vi "CheckVIStatus.vi"() -> ()   [LabVIEW 2016]
panel:
  out "Locked":path[](array[path])=[path "../../../../examples/Open_GDS/GDS/GOOP3_ActiveObject_Debugger_Open_GDS/Map_class/utils/Map_Delete.vi", path "../../../../examples/Open_GDS/GDS/GOOP3_ActiveObject_Debugger_Open_GDS/Map_class/utils/Map_GetAttributes.vi", path "../../../../examples/Open_GDS/GDS/GOOP3_ActiveObject_Debugger_Open_GDS/Map_class/utils/Map_GetAttributesToModify.vi", path "../../../../examples/Open_GDS/GDS/GOOP3_ActiveObject_Debugger_Open_GDS/Map_class/utils/Map_GetClassAttributes.vi", path "../../../../examples/Open_GDS/GDS/GOOP3_ActiveObject_Debugger_Open_GDS/Map_class/utils/Map_GetClassAttributesToModify.vi", path "../../../../examples/Open_GDS/GDS/GOOP3_ActiveObject_Debugger_Open_GDS/Map_class/utils/Map_GetObjectStatus.vi", path "../../../../examples/Open_GDS/GDS/GOOP3_ActiveObject_Debugger_Open_GDS/Map_class/utils/Map_GOOPKernel.vi", path "../../../../examples/Open_GDS/GDS/GOOP3_ActiveObject_Debugger_Open_GDS/Map_class/utils/Map_New.vi", path "../../../../examples/Open_GDS/GDS/GOOP3_ActiveObject_Debugger_Open_GDS/Map_class/utils/Map_SetModifiedAttributes.vi", path "../../../../examples/Open_GDS/GDS/GOOP3_ActiveObject_Debugger_Open_GDS/Map_class/utils/Map_SetModifiedClassAttributes.vi", path "../../../../examples/Open_GDS/GDS/GOOP3_ActiveObject_Debugger_Open_GDS/Object_class/utils/Object_Delete.vi", path "../../../../examples/Open_GDS/GDS/GOOP3_ActiveObject_Debugger_Open_GDS/Object_class/utils/Object_GetAttributes.vi", path "../../../../examples/Open_GDS/GDS/GOOP3_ActiveObject_Debugger_Open_GDS/Object_class/utils/Object_GetAttributesToModify.vi", path "../../../../examples/Open_GDS/GDS/GOOP3_ActiveObject_Debugger_Open_GDS/Object_class/utils/Object_GetClassAttributes.vi", path "../../../../examples/Open_GDS/GDS/GOOP3_ActiveObject_Debugger_Open_GDS/Object_class/utils/Object_GetObjectStatus.vi", path "../../../../examples/Open_GDS/GDS/GOOP3_ActiveObject_Debugger_Open_GDS/Object_class/utils/Object_GOOPKernel.vi", path "../../../../examples/Open_GDS/GDS/GOOP3_ActiveObject_Debugger_Open_GDS/Object_class/utils/Object_New.vi", path "../../../../examples/Open_GDS/GDS/GOOP3_ActiveObject_Debugger_Open_GDS/Object_class/utils/Object_SetModifiedAttributes.vi", path "../../../../examples/Open_GDS/GDS/GOOP3_ActiveObject_Debugger_Open_GDS/Object_class/utils/Object_SetModifiedClassAttributes.vi", path "../../../../examples/Open_GDS/GDS/GOOP4_CreateObjects_Open_GDS/GOOP4_CreateObjects_Open_GDS.aliases", path "../../../../examples/Open_GDS/GDS/GOOP4_CreateObjects_Open_GDS/GOOP4_CreateObjects_Open_GDS.lvlps", path "../../../../examples/Open_GDS/GDS/GOOP4_CreateObjects_Open_GDS/GOOP4_CreateObjects_Open_GDS.lvproj", path "../../../../examples/Open_GDS/GDS/GOOP4_CreateObjects_Open_GDS/GOOP4_Base_class/utils/GOOP4_Base_GetAttributes.vi", path "../../../../examples/Open_GDS/GDS/GOOP4_CreateObjects_Open_GDS/GOOP4_Base_class/utils/GOOP4_Base_New.vi", path "../../../../examples/Open_GDS/GDS/GOOP4_CreateObjects_Open_GDS/GOOP4_Sub_class/utils/GOOP4_Sub_GetAttributes.vi", path "../../../../examples/Open_GDS/GDS/GOOP4_CreateObjects_Open_GDS/GOOP4_Sub_class/utils/GOOP4_Sub_New.vi", path "../../../../examples/Open_GDS/GDS/InterfaceByViServer/InterfaceByViServer.aliases", path "../../../../examples/Open_GDS/GDS/InterfaceByViServer/InterfaceByViServer.lvlps", path "../../../../examples/Open_GDS/GDS/InterfaceByViServer/InterfaceByViServer.lvproj"]
  out "BadVIs":path[](array[path])=[path "../../../../menus/Categories/GOOP.mnu", path "../../../../examples/Open_GDS/Open-GDS.bin3", path "../../../../examples/Open_GDS/GDS/InterfaceByViServer.rar", path "../../../../examples/Open_GDS/GDS/GOOP3_ActiveObject_Debugger_Open_GDS/GOOP3_ActiveObject_Debugger_Open_GDS.aliases", path "../../../../examples/Open_GDS/GDS/GOOP3_ActiveObject_Debugger_Open_GDS/GOOP3_ActiveObject_Debugger_Open_GDS.lvlps", path "../../../../examples/Open_GDS/GDS/GOOP3_ActiveObject_Debugger_Open_GDS/GOOP3_ActiveObject_Debugger_Open_GDS.lvproj", path "../../../../examples/Open_GDS/GDS/GOOP3_ActiveObject_Debugger_Open_GDS/Map_class/Map.lvclass", path "../../../../examples/Open_GDS/GDS/GOOP3_ActiveObject_Debugger_Open_GDS/Object_class/Object.lvclass", path "../../../../examples/Open_GDS/GDS/GOOP4_CreateObjects_Open_GDS/GOOP4_Base_class/GOOP4_Base.lvclass", path "../../../../examples/Open_GDS/GDS/GOOP4_CreateObjects_Open_GDS/GOOP4_Sub_class/GOOP4_Sub.lvclass", path "../../../../examples/Open_GDS/GDS/InterfaceByViServer/Base_class/Base.lvclass", path "../../../../examples/Open_GDS/GDS/InterfaceByViServer/Interface1_Interface/Interface1.lvclass", path "../../../../examples/Open_GDS/GDS/InterfaceByViServer/Leaf_class/Leaf.lvclass", path "../../../../examples/Open_GDS/GDS/InterfaceByViServer/Sub_class/Sub.lvclass", path "../../../../vi.lib/addons/_goop2.llb", path "../../../../vi.lib/addons/_goop3.llb", path "../../../../vi.lib/addons/_goop4.llb", path "../../../../vi.lib/addons/GOOPUtility/dir.mnu", path "../../../../vi.lib/addons/GOOPUtility/GOOPUtility.lvlib", path "../../../../vi.lib/addons/GOOPUtility/_Demo/GOOPUtil_Demo/GOOPUtil Demo ClassDiagram.jpg", path "../../../../vi.lib/addons/GOOPUtility/_Demo/GOOPUtil_Demo/GOOPUtil Demo ClassDiagram.uml", path "../../../../vi.lib/addons/GOOPUtility/_Demo/GOOPUtil_Demo/GOOPUtilDemo.aliases", path "../../../../vi.lib/addons/GOOPUtility/_Demo/GOOPUtil_Demo/GOOPUtilDemo.lvproj", path "../../../../vi.lib/addons/GOOPUtility/_Demo/GOOPUtil_Demo/AnotherClass_class/AnotherClass.lvclass", path "../../../../vi.lib/addons/GOOPUtility/_Demo/GOOPUtil_Demo/DemoClass1_class/DemoClass1.lvclass", path "../../../../vi.lib/addons/GOOPUtility/_Demo/GOOPUtil_Demo/DemoSubClass1_class/DemoSubClass1.lvclass", path "../../../../vi.lib/addons/GOOPUtility/_Demo/GOOPUtil_Demo/DemoSubClass2_class/DemoSubClass2.lvclass", path "../../../../vi.lib/addons/GOOPUtility/_Demo/GOOPUtil_Demo/DemoSubSubClass1_class/DemoSubSubClass1.lvclass", path "Debugger.png", path "GOOP.png", path "OpenGDS.png", path "OpenGDS1.png", path "Thumbs.db", path "UML.png", path "UML_Icon.ico", path "API/API_Description.txt", path "API/GDS_API.mht", path "API/GDSAPI.aliases", path "API/GDSAPI.lvlps", path "API/GDSAPI.lvproj", path "ClassBodyIcons/Actor.png", path "ClassBodyIcons/Interface.png", path "ClassBodyIcons/Message.png", path "ClassProviders/Common/LanguageFiles/en.png", path "ClassProviders/Common/LanguageFiles/gm.png", path "ClassProviders/Common/LanguageFiles/lang_ActorFramework.txt", path "ClassProviders/Common/LanguageFiles/lang_Common.txt", path "ClassProviders/Common/LanguageFiles/lang_Errors.txt", path "ClassProviders/Common/LanguageFiles/lang_IconEditors.txt", path "ClassProviders/Common/LanguageFiles/lang_Installer.txt", path "ClassProviders/Common/LanguageFiles/lang_Licence.txt", path "ClassProviders/Common/LanguageFiles/lang_MainDialogs.txt", path "ClassProviders/Common/LanguageFiles/lang_Menus.txt", path "ClassProviders/Common/LanguageFiles/lang_SignatureDialog.txt", path "ClassProviders/Common/LanguageFiles/lang_StatusMessages.txt", path "ClassProviders/Common/LanguageFiles/lang_UMLTips.txt", path "ClassProviders/Common/LanguageFiles/none.png", path "ClassProviders/Common/LanguageFiles/sv.png", path "ClassProviders/Common/ScriptingFunctions/Scripting.lvclass", path "ClassProviders/CommonClasses/ByViServerInterfaceTemplate_4x4x4/ByViServerInterfaceTemplate_4x4x4.ini", path "ClassProviders/CommonClasses/ByViServerInterfaceTemplate_4x4x4/ByViServerInterfaceTemplate_4x4x4.lvclass", path "ClassProviders/CommonClasses/ByViServerInterfaceTemplate_4x4x4/methods/methods.ini", path "ClassProviders/CommonClasses/ByViServerInterfaceTemplate_6x8x6/ByViServerInterfaceTemplate_6x8x6.ini", path "ClassProviders/CommonClasses/ByViServerInterfaceTemplate_6x8x6/ByViServerInterfaceTemplate_6x8x6.lvclass", path "ClassProviders/CommonClasses/ByViServerInterfaceTemplate_6x8x6/methods/methods.ini", path "ClassProviders/DesignPatterns/ActiveObjects/ActiveObjects_DynamicEvents.ini", path "ClassProviders/DesignPatterns/ActiveObjects/ActiveObjects_QueueQueue.ini", path "ClassProviders/DesignPatterns/ActiveObjects/ActiveObjects_DynamicEvents_SubVIs/ActiveObjects_DynamicEvents_ControlWindow_4x4x4.vi", path "ClassProviders/DesignPatterns/ActiveObjects/ActiveObjects_DynamicEvents_SubVIs/ActiveObjects_DynamicEvents_ControlWindow_4x4x4_Singleton.vi", path "ClassProviders/DesignPatterns/ActiveObjects/ActiveObjects_DynamicEvents_SubVIs/ActiveObjects_DynamicEvents_ControlWindow_6x8x6.vi", path "ClassProviders/DesignPatterns/ActiveObjects/ActiveObjects_DynamicEvents_SubVIs/ActiveObjects_DynamicEvents_ControlWindow_6x8x6_Singleton.vi", path "ClassProviders/DesignPatterns/ActiveObjects/ActiveObjects_DynamicEvents_SubVIs/ActiveObjects_DynamicEvents_Process.vi", path "ClassProviders/DesignPatterns/ActiveObjects/ActiveObjects_DynamicEvents_SubVIs/ActiveObjects_DynamicEvents_ProcessRepository_EndevoGoop3.vi", path "ClassProviders/DesignPatterns/ActiveObjects/ActiveObjects_DynamicEvents_SubVIs/ActiveObjects_DynamicEvents_ProcessRepository_Native.vi", path "ClassProviders/DesignPatterns/ActiveObjects/ActiveObjects_DynamicEvents_SubVIs/ActiveObjects_DynamicEvents_SendMsgToProcess_4x4x4.vi", path "ClassProviders/DesignPatterns/ActiveObjects/ActiveObjects_DynamicEvents_SubVIs/ActiveObjects_DynamicEvents_SendMsgToProcess_4x4x4_Singleton.vi", path "ClassProviders/DesignPatterns/ActiveObjects/ActiveObjects_DynamicEvents_SubVIs/ActiveObjects_DynamicEvents_SendMsgToProcess_6x8x6.vi", path "ClassProviders/DesignPatterns/ActiveObjects/ActiveObjects_DynamicEvents_SubVIs/ActiveObjects_DynamicEvents_SendMsgToProcess_6x8x6_Singleton.vi", path "ClassProviders/DesignPatterns/ActiveObjects/ActiveObjects_DynamicEvents_SubVIs/ActiveObjects_DynamicEvents_StartProcess_OnePerClass.vi", path "ClassProviders/DesignPatterns/ActiveObjects/ActiveObjects_DynamicEvents_SubVIs/ActiveObjects_DynamicEvents_StartProcess_OnePerObject.vi", path "ClassProviders/DesignPatterns/ActiveObjects/ActiveObjects_DynamicEvents_SubVIs/ActiveObjects_DynamicEvents_StopProcess.vi", path "ClassProviders/DesignPatterns/ActiveObjects/ActiveObjects_QueueQueue_SubVIs/ActiveObject_QueueQueue_Process.vi", path "ClassProviders/DesignPatterns/ActiveObjects/ActiveObjects_QueueQueue_SubVIs/ActiveObject_QueueQueue_ProcessRepository_EndevoGoop3.vi", path "ClassProviders/DesignPatterns/ActiveObjects/ActiveObjects_QueueQueue_SubVIs/ActiveObject_QueueQueue_ProcessRepository_Native.vi", path "ClassProviders/DesignPatterns/ActiveObjects/ActiveObjects_QueueQueue_SubVIs/ActiveObject_QueueQueue_StartProcess_OnePerClass.vi", path "ClassProviders/DesignPatterns/ActiveObjects/ActiveObjects_QueueQueue_SubVIs/ActiveObject_QueueQueue_StartProcess_OnePerObject.vi", path "ClassProviders/DesignPatterns/ActiveObjects/ActiveObjects_QueueQueue_SubVIs/ActiveObject_QueueQueue_StopProcess.vi", path "ClassProviders/DesignPatterns/ActiveObjects/ActiveObjects_QueueQueue_SubVIs/ActiveObjects_QueueQueue_SendMsgToProcess_4x4x4.vi", path "ClassProviders/DesignPatterns/ActiveObjects/ActiveObjects_QueueQueue_SubVIs/ActiveObjects_QueueQueue_SendMsgToProcess_4x4x4_Singleton.vi", path "ClassProviders/DesignPatterns/ActiveObjects/ActiveObjects_QueueQueue_SubVIs/ActiveObjects_QueueQueue_SendMsgToProcess_6x8x6.vi", path "ClassProviders/DesignPatterns/ActiveObjects/ActiveObjects_QueueQueue_SubVIs/ActiveObjects_QueueQueue_SendMsgToProcess_6x8x6_Singleton.vi", path "ClassProviders/DesignPatterns/ClassAttributes/ClassAttributes_AddClassAttributes.ini", path "ClassProviders/DesignPatterns/GOOPDebugger/GOOPDebugger_AddDebugging.ini", path "ClassProviders/DesignPatterns/GOOPDebugger/GOOPDebugger_SubVIs/GOOPDebugger_GetObjectStatus_4x4x4.vi", path "ClassProviders/DesignPatterns/GOOPDebugger/GOOPDebugger_SubVIs/GOOPDebugger_GetObjectStatus_6x8x6.vi", path "ClassProviders/DesignPatterns/Interface/Interface_ImplementInterface.ini", path "ClassProviders/DesignPatterns/Interface/Interface_SubVIs/Interface_GetReference_4x4x4.vi", path "ClassProviders/DesignPatterns/Interface/Interface_SubVIs/Interface_GetReference_6x8x6.vi", path "ClassProviders/DesignPatterns/Interface/Interface_SubVIs/Interface_Implement.vi", path "ClassProviders/DesignPatterns/Persistent/Persistent_MakePersistent.ini", path "ClassProviders/DesignPatterns/Persistent/Persistent_SubVIs/Persistent_CreateReference_4x4x4.vi", path "ClassProviders/DesignPatterns/Persistent/Persistent_SubVIs/Persistent_CreateReference_6x8x6.vi", path "ClassProviders/DesignPatterns/Persistent/Persistent_SubVIs/Persistent_New_4x4x4.vi", path "ClassProviders/DesignPatterns/Persistent/Persistent_SubVIs/Persistent_New_6x8x6.vi", path "ClassProviders/DesignPatterns/ReferencedVariables/ReferencedVariables_AddReferenceVariable.ini", path "ClassProviders/DesignPatterns/ReferencedVariables/ReferencedVariables_SubVIs/ReferencedVariables_CreateReferenceVariable_4x4x4.vi", path "ClassProviders/DesignPatterns/ReferencedVariables/ReferencedVariables_SubVIs/ReferencedVariables_CreateReferenceVariable_6x8x6.vi", path "ClassProviders/DesignPatterns/ReferencedVariables/ReferencedVariables_SubVIs/ReferencedVariables_DeleteReferenceVariable_4x4x4.vi", path "ClassProviders/DesignPatterns/ReferencedVariables/ReferencedVariables_SubVIs/ReferencedVariables_DeleteReferenceVariable_6x8x6.vi", path "ClassProviders/DesignPatterns/ReferencedVariables/ReferencedVariables_SubVIs/ReferencedVariables_ReadReferencedVariable_4x4x4.vi", path "ClassProviders/DesignPatterns/ReferencedVariables/ReferencedVariables_SubVIs/ReferencedVariables_ReadReferencedVariable_4x4x4_Singleton.vi", path "ClassProviders/DesignPatterns/ReferencedVariables/ReferencedVariables_SubVIs/ReferencedVariables_ReadReferencedVariable_6x8x6.vi", path "ClassProviders/DesignPatterns/ReferencedVariables/ReferencedVariables_SubVIs/ReferencedVariables_ReadReferencedVariable_6x8x6_Singleton.vi", path "ClassProviders/DesignPatterns/ReferencedVariables/ReferencedVariables_SubVIs/ReferencedVariables_ReadWriteReferencedVariable_4x4x4.vi", path "ClassProviders/DesignPatterns/ReferencedVariables/ReferencedVariables_SubVIs/ReferencedVariables_ReadWriteReferencedVariable_4x4x4_Singleton.vi", path "ClassProviders/DesignPatterns/ReferencedVariables/ReferencedVariables_SubVIs/ReferencedVariables_ReadWriteReferencedVariable_6x8x6.vi", path "ClassProviders/DesignPatterns/ReferencedVariables/ReferencedVariables_SubVIs/ReferencedVariables_ReadWriteReferencedVariable_6x8x6_Singleton.vi", path "ClassProviders/Provider_BaseClassInterface/ClassReader_class/ClassReader.lvclass", path "ClassProviders/Provider_BaseClassInterface/ClassWriter_class/ClassWriter.lvclass", path "ClassProviders/Provider_EndevoGOOP300/ClassReaderGOOP300_class/ClassReaderGOOP300.lvclass", path "ClassProviders/Provider_EndevoGOOP300/ClassWriterGOOP300_class/ClassWriterGOOP300.lvclass", path "ClassProviders/Provider_EndevoGOOP300/Templates/TemplateProjects.aliases", path "ClassProviders/Provider_EndevoGOOP300/Templates/TemplateProjects.lvlps", path "ClassProviders/Provider_EndevoGOOP300/Templates/TemplateProjects.lvproj", path "ClassProviders/Provider_EndevoGOOP300/Templates/BaseTemplate/BaseTemplate.lvclass", path "ClassProviders/Provider_EndevoGOOP300/Templates/BaseTemplate/methods/B_GetProperty.vi", path "ClassProviders/Provider_EndevoGOOP300/Templates/BaseTemplate/methods/B_NoneModifing.vi", path "ClassProviders/Provider_EndevoGOOP300/Templates/BaseTemplate/methods/B_ReadAttribute.vi", path "ClassProviders/Provider_EndevoGOOP300/Templates/BaseTemplate/methods/B_ReadClassAttribute.vi", path "ClassProviders/Provider_EndevoGOOP300/Templates/BaseTemplate/methods/B_ReadProperty.vi", path "ClassProviders/Provider_EndevoGOOP300/Templates/BaseTemplate/methods/B_ReadWriteAttribute.vi", path "ClassProviders/Provider_EndevoGOOP300/Templates/BaseTemplate/methods/B_ReadWriteClassAttribute.vi", path "ClassProviders/Provider_EndevoGOOP300/Templates/BaseTemplate/methods/B_SetProperty.vi", path "ClassProviders/Provider_EndevoGOOP300/Templates/BaseTemplate/methods/B_WriteAttribute.vi", path "ClassProviders/Provider_EndevoGOOP300/Templates/BaseTemplate/methods/B_WriteClassAttribute.vi", path "ClassProviders/Provider_EndevoGOOP300/Templates/BaseTemplate/methods/B_WriteProperty.vi", path "ClassProviders/Provider_EndevoGOOP300/Templates/BaseTemplate/methods/methods.ini", path "ClassProviders/Provider_EndevoGOOP300/Templates/BaseTemplate/utils/vssver.scc", path "ClassProviders/Provider_EndevoGOOP300/Templates/BaseTemplate_4x4x4/BaseTemplate_4x4x4.lvclass", path "ClassProviders/Provider_EndevoGOOP300/Templates/BaseTemplate_4x4x4/methods/methods.ini", path "ClassProviders/Provider_EndevoGOOP300/Templates/SingletonTemplate/SingletonTemplate.lvclass", path "ClassProviders/Provider_EndevoGOOP300/Templates/SingletonTemplate/methods/methods.ini", path "ClassProviders/Provider_EndevoGOOP300/Templates/SingletonTemplate/methods/Sgl_GetProperty.vi", path "ClassProviders/Provider_EndevoGOOP300/Templates/SingletonTemplate/methods/Sgl_NoneModifing.vi", path "ClassProviders/Provider_EndevoGOOP300/Templates/SingletonTemplate/methods/Sgl_ReadAttribute.vi", path "ClassProviders/Provider_EndevoGOOP300/Templates/SingletonTemplate/methods/Sgl_ReadWriteAttribute.vi", path "ClassProviders/Provider_EndevoGOOP300/Templates/SingletonTemplate/methods/Sgl_SetProperty.vi", path "ClassProviders/Provider_EndevoGOOP300/Templates/SingletonTemplate/methods/Sgl_WriteAttribute.vi", path "ClassProviders/Provider_EndevoGOOP300/Templates/SubTemplate/SubTemplate.lvclass", path "ClassProviders/Provider_EndevoGOOP300/Templates/SubTemplate/methods/methods.ini", path "ClassProviders/Provider_EndevoGOOP300/Templates/SubTemplate_4x4x4/SubTemplate_4x4x4.lvclass", path "ClassProviders/Provider_EndevoGOOP300/Templates/SubTemplate_4x4x4/methods/methods.ini", path "ClassProviders/Provider_EndevoGOOP400/Templates.rar", path "ClassProviders/Provider_EndevoGOOP400/ClassReaderGOOP400_class/ClassReaderGOOP400.lvclass", path "ClassProviders/Provider_EndevoGOOP400/ClassWriterGOOP400_class/ClassWriterGOOP400.lvclass", path "ClassProviders/Provider_EndevoGOOP400/Templates/G4Template.aliases", path "ClassProviders/Provider_EndevoGOOP400/Templates/G4Template.lvproj", path "ClassProviders/Provider_EndevoGOOP400/Templates/G4BaseTemplate_Simple_4x4x4/G4BaseTemplate_Simple_4x4x4.lvclass", path "ClassProviders/Provider_EndevoGOOP400/Templates/G4BaseTemplate_Simple_4x4x4/methods/G4BaseTemplate_Simple_4x4x4_GetProperty.vi", path "ClassProviders/Provider_EndevoGOOP400/Templates/G4BaseTemplate_Simple_4x4x4/methods/G4BaseTemplate_Simple_4x4x4_NoneModifing.vi", path "ClassProviders/Provider_EndevoGOOP400/Templates/G4BaseTemplate_Simple_4x4x4/methods/G4BaseTemplate_Simple_4x4x4_ReadAttribute.vi", path "ClassProviders/Provider_EndevoGOOP400/Templates/G4BaseTemplate_Simple_4x4x4/methods/G4BaseTemplate_Simple_4x4x4_ReadProperty.vi", path "ClassProviders/Provider_EndevoGOOP400/Templates/G4BaseTemplate_Simple_4x4x4/methods/G4BaseTemplate_Simple_4x4x4_ReadWriteAttribute.vi", path "ClassProviders/Provider_EndevoGOOP400/Templates/G4BaseTemplate_Simple_4x4x4/methods/G4BaseTemplate_Simple_4x4x4_SetProperty.vi", path "ClassProviders/Provider_EndevoGOOP400/Templates/G4BaseTemplate_Simple_4x4x4/methods/G4BaseTemplate_Simple_4x4x4_WriteAttribute.vi", path "ClassProviders/Provider_EndevoGOOP400/Templates/G4BaseTemplate_Simple_4x4x4/methods/G4BaseTemplate_Simple_4x4x4_WriteProperty.vi", path "ClassProviders/Provider_EndevoGOOP400/Templates/G4BaseTemplate_Simple_4x4x4/methods/methods.ini", path "ClassProviders/Provider_EndevoGOOP400/Templates/G4BaseTemplate_Simple_6x8x6/G4BaseTemplate_Simple_6x8x6.lvclass", path "ClassProviders/Provider_EndevoGOOP400/Templates/G4BaseTemplate_Simple_6x8x6/methods/G4BaseTemplate_Simple_6x8x6_GetProperty.vi", path "ClassProviders/Provider_EndevoGOOP400/Templates/G4BaseTemplate_Simple_6x8x6/methods/G4BaseTemplate_Simple_6x8x6_NoneModifing.vi", path "ClassProviders/Provider_EndevoGOOP400/Templates/G4BaseTemplate_Simple_6x8x6/methods/G4BaseTemplate_Simple_6x8x6_ReadAttribute.vi", path "ClassProviders/Provider_EndevoGOOP400/Templates/G4BaseTemplate_Simple_6x8x6/methods/G4BaseTemplate_Simple_6x8x6_ReadProperty.vi", path "ClassProviders/Provider_EndevoGOOP400/Templates/G4BaseTemplate_Simple_6x8x6/methods/G4BaseTemplate_Simple_6x8x6_ReadWriteAttribute.vi", path "ClassProviders/Provider_EndevoGOOP400/Templates/G4BaseTemplate_Simple_6x8x6/methods/G4BaseTemplate_Simple_6x8x6_SetProperty.vi", path "ClassProviders/Provider_EndevoGOOP400/Templates/G4BaseTemplate_Simple_6x8x6/methods/G4BaseTemplate_Simple_6x8x6_WriteAttribute.vi", path "ClassProviders/Provider_EndevoGOOP400/Templates/G4BaseTemplate_Simple_6x8x6/methods/G4BaseTemplate_Simple_6x8x6_WriteProperty.vi", path "ClassProviders/Provider_EndevoGOOP400/Templates/G4BaseTemplate_Simple_6x8x6/methods/methods.ini", path "ClassProviders/Provider_EndevoGOOP400/Templates/G4BaseTemplate_Singleton_4x4x4/G4BaseTemplate_Singleton_4x4x4.lvclass", path "ClassProviders/Provider_EndevoGOOP400/Templates/G4BaseTemplate_Singleton_4x4x4/methods/G4BaseTemplate_Singleton_4x4x4_GetProperty.vi", path "ClassProviders/Provider_EndevoGOOP400/Templates/G4BaseTemplate_Singleton_4x4x4/methods/G4BaseTemplate_Singleton_4x4x4_ReadAttribute.vi", path "ClassProviders/Provider_EndevoGOOP400/Templates/G4BaseTemplate_Singleton_4x4x4/methods/G4BaseTemplate_Singleton_4x4x4_ReadWriteAttribute.vi", path "ClassProviders/Provider_EndevoGOOP400/Templates/G4BaseTemplate_Singleton_4x4x4/methods/G4BaseTemplate_Singleton_4x4x4_SetProperty.vi", path "ClassProviders/Provider_EndevoGOOP400/Templates/G4BaseTemplate_Singleton_4x4x4/methods/G4BaseTemplate_Singleton_4x4x4_WriteAttribute.vi", path "ClassProviders/Provider_EndevoGOOP400/Templates/G4BaseTemplate_Singleton_4x4x4/methods/methods.ini", path "ClassProviders/Provider_EndevoGOOP400/Templates/G4BaseTemplate_Singleton_4x4x4/methods/methods.txt", path "ClassProviders/Provider_EndevoGOOP400/Templates/G4BaseTemplate_Singleton_6x8x6/G4BaseTemplate_Singleton_6x8x6.lvclass", path "ClassProviders/Provider_EndevoGOOP400/Templates/G4BaseTemplate_Singleton_6x8x6/methods/G4BaseTemplate_Singleton_6x8x6_GetProperty.vi", path "ClassProviders/Provider_EndevoGOOP400/Templates/G4BaseTemplate_Singleton_6x8x6/methods/G4BaseTemplate_Singleton_6x8x6_ReadAttribute.vi", path "ClassProviders/Provider_EndevoGOOP400/Templates/G4BaseTemplate_Singleton_6x8x6/methods/G4BaseTemplate_Singleton_6x8x6_ReadWriteAttribute.vi", path "ClassProviders/Provider_EndevoGOOP400/Templates/G4BaseTemplate_Singleton_6x8x6/methods/G4BaseTemplate_Singleton_6x8x6_SetProperty.vi", path "ClassProviders/Provider_EndevoGOOP400/Templates/G4BaseTemplate_Singleton_6x8x6/methods/G4BaseTemplate_Singleton_6x8x6_WriteAttribute.vi", path "ClassProviders/Provider_EndevoGOOP400/Templates/G4BaseTemplate_Singleton_6x8x6/methods/methods.ini", path "ClassProviders/Provider_EndevoGOOP400/Templates/G4InterfaceTemplate_4x4x4/G4InterfaceTemplate_4x4x4.ini", path "ClassProviders/Provider_EndevoGOOP400/Templates/G4InterfaceTemplate_4x4x4/G4InterfaceTemplate_4x4x4.lvclass", path "ClassProviders/Provider_EndevoGOOP400/Templates/G4InterfaceTemplate_4x4x4/methods/G4InterfaceTemplate_4x4x4_Method.vi", path "ClassProviders/Provider_EndevoGOOP400/Templates/G4InterfaceTemplate_4x4x4/methods/methods.ini", path "ClassProviders/Provider_EndevoGOOP400/Templates/G4InterfaceTemplate_6x8x6/G4InterfaceTemplate_6x8x6.ini", path "ClassProviders/Provider_EndevoGOOP400/Templates/G4InterfaceTemplate_6x8x6/G4InterfaceTemplate_6x8x6.lvclass", path "ClassProviders/Provider_EndevoGOOP400/Templates/G4InterfaceTemplate_6x8x6/methods/G4InterfaceTemplate_6x8x6_Method.vi", path "ClassProviders/Provider_EndevoGOOP400/Templates/G4InterfaceTemplate_6x8x6/methods/methods.ini", path "ClassProviders/Provider_EndevoGOOP400/Templates/G4SubTemplate_Simple_4x4x4/G4SubTemplate_Simple_4x4x4.lvclass", path "ClassProviders/Provider_EndevoGOOP400/Templates/G4SubTemplate_Simple_4x4x4/methods/G4SubTemplate_Simple_4x4x4_GetProperty.vi", path "ClassProviders/Provider_EndevoGOOP400/Templates/G4SubTemplate_Simple_4x4x4/methods/G4SubTemplate_Simple_4x4x4_NoneModifing.vi", path "ClassProviders/Provider_EndevoGOOP400/Templates/G4SubTemplate_Simple_4x4x4/methods/G4SubTemplate_Simple_4x4x4_ReadAttribute.vi", path "ClassProviders/Provider_EndevoGOOP400/Templates/G4SubTemplate_Simple_4x4x4/methods/G4SubTemplate_Simple_4x4x4_ReadProperty.vi", path "ClassProviders/Provider_EndevoGOOP400/Templates/G4SubTemplate_Simple_4x4x4/methods/G4SubTemplate_Simple_4x4x4_ReadWriteAttribute.vi", path "ClassProviders/Provider_EndevoGOOP400/Templates/G4SubTemplate_Simple_4x4x4/methods/G4SubTemplate_Simple_4x4x4_SetProperty.vi", path "ClassProviders/Provider_EndevoGOOP400/Templates/G4SubTemplate_Simple_4x4x4/methods/G4SubTemplate_Simple_4x4x4_WriteAttribute.vi", path "ClassProviders/Provider_EndevoGOOP400/Templates/G4SubTemplate_Simple_4x4x4/methods/G4SubTemplate_Simple_4x4x4_WriteProperty.vi", path "ClassProviders/Provider_EndevoGOOP400/Templates/G4SubTemplate_Simple_4x4x4/methods/methods.ini", path "ClassProviders/Provider_EndevoGOOP400/Templates/G4SubTemplate_Simple_6x8x6/G4SubTemplate_Simple_6x8x6.lvclass", path "ClassProviders/Provider_EndevoGOOP400/Templates/G4SubTemplate_Simple_6x8x6/methods/G4SubTemplate_Simple_6x8x6_GetProperty.vi", path "ClassProviders/Provider_EndevoGOOP400/Templates/G4SubTemplate_Simple_6x8x6/methods/G4SubTemplate_Simple_6x8x6_NoneModifing.vi", path "ClassProviders/Provider_EndevoGOOP400/Templates/G4SubTemplate_Simple_6x8x6/methods/G4SubTemplate_Simple_6x8x6_ReadAttribute.vi", path "ClassProviders/Provider_EndevoGOOP400/Templates/G4SubTemplate_Simple_6x8x6/methods/G4SubTemplate_Simple_6x8x6_ReadProperty.vi", path "ClassProviders/Provider_EndevoGOOP400/Templates/G4SubTemplate_Simple_6x8x6/methods/G4SubTemplate_Simple_6x8x6_ReadWriteAttribute.vi", path "ClassProviders/Provider_EndevoGOOP400/Templates/G4SubTemplate_Simple_6x8x6/methods/G4SubTemplate_Simple_6x8x6_SetProperty.vi", path "ClassProviders/Provider_EndevoGOOP400/Templates/G4SubTemplate_Simple_6x8x6/methods/G4SubTemplate_Simple_6x8x6_WriteAttribute.vi", path "ClassProviders/Provider_EndevoGOOP400/Templates/G4SubTemplate_Simple_6x8x6/methods/G4SubTemplate_Simple_6x8x6_WriteProperty.vi", path "ClassProviders/Provider_EndevoGOOP400/Templates/G4SubTemplate_Simple_6x8x6/methods/methods.ini", path "ClassProviders/Provider_EndevoGOOP400/Templates/G4SubTemplate_Singleton_4x4x4/G4SubTemplate_Singleton_4x4x4.lvclass", path "ClassProviders/Provider_EndevoGOOP400/Templates/G4SubTemplate_Singleton_4x4x4/methods/G4SubTemplate_Singleton_4x4x4_GetProperty.vi", path "ClassProviders/Provider_EndevoGOOP400/Templates/G4SubTemplate_Singleton_4x4x4/methods/G4SubTemplate_Singleton_4x4x4_ReadAttribute.vi", path "ClassProviders/Provider_EndevoGOOP400/Templates/G4SubTemplate_Singleton_4x4x4/methods/G4SubTemplate_Singleton_4x4x4_ReadWriteAttribute.vi", path "ClassProviders/Provider_EndevoGOOP400/Templates/G4SubTemplate_Singleton_4x4x4/methods/G4SubTemplate_Singleton_4x4x4_SetProperty.vi", path "ClassProviders/Provider_EndevoGOOP400/Templates/G4SubTemplate_Singleton_4x4x4/methods/G4SubTemplate_Singleton_4x4x4_WriteAttribute.vi", path "ClassProviders/Provider_EndevoGOOP400/Templates/G4SubTemplate_Singleton_4x4x4/methods/methods.ini", path "ClassProviders/Provider_EndevoGOOP400/Templates/G4SubTemplate_Singleton_6x8x6/G4SubTemplate_Singleton_6x8x6.lvclass", path "ClassProviders/Provider_EndevoGOOP400/Templates/G4SubTemplate_Singleton_6x8x6/methods/G4SubTemplate_Singleton_6x8x6_GetProperty.vi", path "ClassProviders/Provider_EndevoGOOP400/Templates/G4SubTemplate_Singleton_6x8x6/methods/G4SubTemplate_Singleton_6x8x6_ReadAttribute.vi", path "ClassProviders/Provider_EndevoGOOP400/Templates/G4SubTemplate_Singleton_6x8x6/methods/G4SubTemplate_Singleton_6x8x6_ReadWriteAttribute.vi", path "ClassProviders/Provider_EndevoGOOP400/Templates/G4SubTemplate_Singleton_6x8x6/methods/G4SubTemplate_Singleton_6x8x6_SetProperty.vi", path "ClassProviders/Provider_EndevoGOOP400/Templates/G4SubTemplate_Singleton_6x8x6/methods/G4SubTemplate_Singleton_6x8x6_WriteAttribute.vi", path "ClassProviders/Provider_EndevoGOOP400/Templates/G4SubTemplate_Singleton_6x8x6/methods/methods.ini", path "ClassProviders/Provider_LvNativeClass/ClassReaderNative_class/ClassReaderNative.lvclass", path "ClassProviders/Provider_LvNativeClass/ClassWriterNative_class/ClassWriterNative.lvclass", path "ClassProviders/Provider_LvNativeClass/Templates/NativeBaseTemplate/NativeBaseTemplate.lvclass", path "ClassProviders/Provider_LvNativeClass/Templates/NativeBaseTemplate/methods/methods.ini", path "ClassProviders/Provider_LvNativeClass/Templates/NativeBaseTemplate_4x4x4/NativeBaseTemplate_4x4x4.lvclass", path "ClassProviders/Provider_LvNativeClass/Templates/NativeBaseTemplate_4x4x4/methods/methods.ini", path "ClassProviders/Provider_LvNativeClass/Templates/NativeSubTemplate/NativeSubTemplate.lvclass", path "ClassProviders/Provider_LvNativeClass/Templates/NativeSubTemplate/methods/methods.ini", path "ClassProviders/Provider_LvNativeClass/Templates/NativeSubTemplate_4x4x4/NativeSubTemplate_4x4x4.lvclass", path "ClassProviders/Provider_LvNativeClass/Templates/NativeSubTemplate_4x4x4/methods/methods.ini", path "ClassProviders/StaticMethods/methods.ini", path "Glyphs/Actor.png", path "Glyphs/ActorCore.png", path "Glyphs/Application.png", path "Glyphs/Do.png", path "Glyphs/Emergency.png", path "Glyphs/Interface.png", path "Glyphs/LaunchActor.png", path "Glyphs/Load.png", path "Glyphs/Log.png", path "Glyphs/Mail.png", path "Glyphs/MessageClass.png", path "Glyphs/SendTask.png", path "Glyphs/Stop.png", path "HelpFiles/OpenGDS_GOOPHelp.htm", path "HelpFiles/files/ChangeorAddMethodsinaClassTemp5.html", path "HelpFiles/files/ClassDiagram5.html", path "HelpFiles/files/CreateClassTemplate5.html", path "HelpFiles/files/CreateDesignPattern5.html", path "HelpFiles/files/CreateNewClass5.html", path "HelpFiles/files/CreateNewMethod5.html", path "HelpFiles/files/CreateVIIcon5.html", path "HelpFiles/files/Demos5.html", path "HelpFiles/files/EndevoGOOP3ClassTemplate5.html", path "HelpFiles/files/EndevoGOOP4ClassTemplate5.html", path "HelpFiles/files/file.gif", path "HelpFiles/files/Findingthefeatures5.html", path "HelpFiles/files/folder-closed.gif", path "HelpFiles/files/folder.gif", path "HelpFiles/files/GettingStartedwithGOOPDevelopm5.html", path "HelpFiles/files/GOOP4vsGOOP35.html", path "HelpFiles/files/GOOPDebugger5.html", path "HelpFiles/files/GOOPOptionsDialog5.html", path "HelpFiles/files/hnd.css", path "HelpFiles/files/hnd.js", path "HelpFiles/files/HowGOOP3comparestoGOOP25.html", path "HelpFiles/files/img_1.jpg", path "HelpFiles/files/img_1.png", path "HelpFiles/files/img_10.jpg", path "HelpFiles/files/img_10.png", path "HelpFiles/files/img_11.png", path "HelpFiles/files/img_111.jpg", path "HelpFiles/files/img_114.jpg", path "HelpFiles/files/img_116.jpg", path "HelpFiles/files/img_118.jpg", path "HelpFiles/files/img_12.png", path "HelpFiles/files/img_125.jpg", path "HelpFiles/files/img_13.png", path "HelpFiles/files/img_138.jpg", path "HelpFiles/files/img_14.png", path "HelpFiles/files/img_141.jpg", path "HelpFiles/files/img_143.jpg", path "HelpFiles/files/img_145.jpg", path "HelpFiles/files/img_15.png", path "HelpFiles/files/img_152.jpg", path "HelpFiles/files/img_16.png", path "HelpFiles/files/img_17.jpg", path "HelpFiles/files/img_17.png", path "HelpFiles/files/img_18.png", path "HelpFiles/files/img_19.png", path "HelpFiles/files/img_2.png", path "HelpFiles/files/img_20.png", path "HelpFiles/files/img_21.png", path "HelpFiles/files/img_22.png", path "HelpFiles/files/img_23.png", path "HelpFiles/files/img_24.png", path "HelpFiles/files/img_25.png", path "HelpFiles/files/img_26.png", path "HelpFiles/files/img_27.png", path "HelpFiles/files/img_28.png", path "HelpFiles/files/img_29.png", path "HelpFiles/files/img_3.jpg", path "HelpFiles/files/img_3.png", path "HelpFiles/files/img_30.jpg", path "HelpFiles/files/img_30.png", path "HelpFiles/files/img_33.jpg", path "HelpFiles/files/img_35.jpg", path "HelpFiles/files/img_37.jpg", path "HelpFiles/files/img_4.png", path "HelpFiles/files/img_44.jpg", path "HelpFiles/files/img_5.png", path "HelpFiles/files/img_57.jpg", path "HelpFiles/files/img_6.jpg", path "HelpFiles/files/img_6.png", path "HelpFiles/files/img_60.jpg", path "HelpFiles/files/img_62.jpg", path "HelpFiles/files/img_64.jpg", path "HelpFiles/files/img_7.png", path "HelpFiles/files/img_71.jpg", path "HelpFiles/files/img_8.jpg", path "HelpFiles/files/img_8.png", path "HelpFiles/files/img_84.jpg", path "HelpFiles/files/img_87.jpg", path "HelpFiles/files/img_89.jpg", path "HelpFiles/files/img_9.png", path "HelpFiles/files/img_91.jpg", path "HelpFiles/files/img_98.jpg", path "HelpFiles/files/jquery.cookie.js", path "HelpFiles/files/jquery.min.js", path "HelpFiles/files/jquery.rich-array-hnd.js", path "HelpFiles/files/jquery.treeview.min.js", path "HelpFiles/files/jsrelative.js", path "HelpFiles/files/minus.gif", path "HelpFiles/files/PackageDiagram5.html", path "HelpFiles/files/PlatformCompatibility.html", path "HelpFiles/files/plus.gif", path "HelpFiles/files/searchdata.js", path "HelpFiles/files/SequenceDiagram5.html", path "HelpFiles/files/StateDiagram5.html", path "HelpFiles/files/toc.css", path "HelpFiles/files/toc.htm", path "HelpFiles/files/treeview-black-line.gif", path "HelpFiles/files/treeview-black.gif", path "HelpFiles/files/treeview-default-line.gif", path "HelpFiles/files/treeview-default.gif", path "HelpFiles/files/treeview-famfamfam-line.gif", path "HelpFiles/files/treeview-famfamfam.gif", path "HelpFiles/files/treeview-gray-line.gif", path "HelpFiles/files/treeview-gray.gif", path "HelpFiles/files/treeview-red-line.gif", path "HelpFiles/files/treeview-red.gif", path "HelpFiles/files/UMLModeller5.html", path "HelpFiles/files/UseCaseDiagram5.html", path "Icons/_VirtualFolder_Messages.png", path "Icons/BlueCircle.png", path "Icons/BlueFrame.PNG", path "Icons/BlueFull.PNG", path "Icons/BlueMessage.png", path "Icons/BrownCircle.png", path "Icons/BrownFrame.png", path "Icons/BrownFull.png", path "Icons/BurgundyCircle.png", path "Icons/BurgundyFrame.png", path "Icons/BurgundyFull.png", path "Icons/CyanCircle.png", path "Icons/CyanFrame.png", path "Icons/CyanFull.png", path "Icons/DarkBlueCircle.png", path "Icons/DarkBlueFrame.png", path "Icons/DarkBlueFull.png", path "Icons/ForestGreenCircle.png", path "Icons/ForestGreenFrame.png", path "Icons/ForestGreenFull.png", path "Icons/GrayCircle.PNG", path "Icons/GrayFrame.PNG", path "Icons/GrayFull.PNG", path "Icons/GreenCircle.png", path "Icons/GreenFrame.png", path "Icons/GreenFull.png", path "Icons/Interface.png", path "Icons/LightGreenCircle.png", path "Icons/LightGreenFrame.png", path "Icons/LightGreenFull.png", path "Icons/LightRedCircle.png", path "Icons/LightRedFrame.png", path "Icons/LightRedFull.png", path "Icons/PinkCircle.png", path "Icons/PinkFrame.png", path "Icons/PinkFull.png", path "Icons/PurpleCircle.png", path "Icons/PurpleFrame.png", path "Icons/PurpleFull.png", path "Icons/RedCircle.png", path "Icons/RedFrame.png", path "Icons/RedFull.PNG", path "Icons/Thumbs.db", path "Icons/YellowCircle.PNG", path "Icons/YellowFrame.png", path "Icons/YellowFull.png", path "UML/UMLEditor.rtm", path "UML/AbstractEdge_class/AbstractEdge.lvclass", path "UML/AbstractNode_class/AbstractNode.lvclass", path "UML/ActorNode_class/ActorNode.lvclass", path "UML/ArrowHead_class/ArrowHead.lvclass", path "UML/BentStyle_class/BentStyle.lvclass", path "UML/CallEdge_class/CallEdge.lvclass", path "UML/CallNode_class/CallNode.lvclass", path "UML/ClassDiagramGraph_class/ClassDiagramGraph.lvclass", path "UML/ClassNode_class/ClassNode.lvclass", path "UML/ClassRelationshipEdge_class/ClassRelationshipEdge.lvclass", path "UML/DesignPattern/DesignPatterns/AbstractFactory.xml", path "UML/DesignPattern/DesignPatterns/Adapter.xml", path "UML/DesignPattern/DesignPatterns/Bridge.xml", path "UML/DesignPattern/DesignPatterns/Builder.xml", path "UML/DesignPattern/DesignPatterns/ChainofResponsibility.xml", path "UML/DesignPattern/DesignPatterns/Command.xml", path "UML/DesignPattern/DesignPatterns/Composite.xml", path "UML/DesignPattern/DesignPatterns/Decorator.xml", path "UML/DesignPattern/DesignPatterns/Facade.xml", path "UML/DesignPattern/DesignPatterns/FactoryMethod.xml", path "UML/DesignPattern/DesignPatterns/Flyweight.xml", path "UML/DesignPattern/DesignPatterns/Interpreter.xml", path "UML/DesignPattern/DesignPatterns/Iterator.xml", path "UML/DesignPattern/DesignPatterns/Mediator.xml", path "UML/DesignPattern/DesignPatterns/Memento.xml", path "UML/DesignPattern/DesignPatterns/Observer.xml", path "UML/DesignPattern/DesignPatterns/Prototype.xml", path "UML/DesignPattern/DesignPatterns/Proxy.xml", path "UML/DesignPattern/DesignPatterns/Singleton.xml", path "UML/DesignPattern/DesignPatterns/State.xml", path "UML/DesignPattern/DesignPatterns/Strategy.xml", path "UML/DesignPattern/DesignPatterns/TemplateMethod.xml", path "UML/DesignPattern/DesignPatterns/Visitor.xml", path "UML/Direction_class/Direction.lvclass", path "UML/FinalStateNode_class/FinalStateNode.lvclass", path "UML/GeneralPathEdge_class/GeneralPathEdge.lvclass", path "UML/Graph_class/Graph.lvclass", path "UML/Graphics_class/Graphics.lvclass", path "UML/Grid_class/Grid.lvclass", path "UML/ImplicitParameterNode_class/ImplicitParameterNode.lvclass", path "UML/InitialStateNode_class/InitialStateNode.lvclass", path "UML/InterfaceNode_class/InterfaceNode.lvclass", path "UML/LineStyle_class/LineStyle.lvclass", path "UML/MultiLineString_class/MultiLineString.lvclass", path "UML/NoteEdge_class/NoteEdge.lvclass", path "UML/NoteNode_class/NoteNode.lvclass", path "UML/PackageNode_class/PackageNode.lvclass", path "UML/PointNode_class/PointNode.lvclass", path "UML/RectangularNode_class/RectangularNode.lvclass", path "UML/SegmentedLineEdge_class/SegmentedLineEdge.lvclass", path "UML/SequenceDiagramGraph_class/SequenceDiagramGraph.lvclass", path "UML/StateDiagramGraph_class/StateDiagramGraph.lvclass", path "UML/StateNode_class/StateNode.lvclass", path "UML/StateReverse_class/StateReverse.lvclass", path "UML/StateTransitionEdge_class/StateTransitionEdge.lvclass", path "UML/SystemNode_class/SystemNode.lvclass", path "UML/UmlEditor_class/UmlEditor.lvclass", path "UML/UseCaseDiagramGraph_class/UseCaseDiagramGraph.lvclass", path "UML/UseCaseNode_class/UseCaseNode.lvclass", path "UmlMessage/UmlMessage_Folder.txt", path "UmlMessage/UmlMessager_2012-64.exe", path "UmlMessage/UmlMessager_2012.exe", path "UmlMessage/UmlMessager_2013-64.exe", path "UmlMessage/UmlMessager_2013.exe", path "UmlMessage/UmlMessager_2014-64.exe", path "UmlMessage/UmlMessager_2014.exe", path "UmlMessage/UmlMessager_2015.exe", path "../GProviders/GOOP_Library.ini", path "../GProviders/GOOP_LVClass.ini", path "../GProviders/GOOP_MyComputer.ini", path "../GProviders/GOOP_VI.ini", path "../GProviders/GOOP_VirtualFolder.ini", path "../GProviders/GOOP_XControl.ini"]
  out "Modified":path[](array[path])=[path "ClassProviders/Common/File/File_FileInfo.ctl", path "ClassProviders/Common/ScriptingFunctions/Scripting_BundleByName.vi", path "ClassProviders/Common/ScriptingFunctions/Scripting_G1DeleteToG3Delete.vi", path "ClassProviders/Common/ScriptingFunctions/Scripting_G1NewToG3New.vi", path "ClassProviders/Common/ScriptingFunctions/Scripting_GetStateMachineReferences.vi", path "ClassProviders/Common/ScriptingFunctions/Scripting_LVClassScriptingProps.vi", path "ClassProviders/Common/ScriptingFunctions/Scripting_PlaceDVRRefInClassAttribute.vi", path "ClassProviders/Common/ScriptingFunctions/Scripting_UnBundleByName.vi", path "ClassProviders/Provider_EndevoGOOP300/Templates/BaseTemplate_4x4x4/methods/B_GetProperty.vi", path "ClassProviders/Provider_EndevoGOOP300/Templates/BaseTemplate_4x4x4/methods/B_NoneModifing.vi", path "ClassProviders/Provider_EndevoGOOP300/Templates/BaseTemplate_4x4x4/methods/B_ReadAttribute.vi", path "ClassProviders/Provider_EndevoGOOP300/Templates/BaseTemplate_4x4x4/methods/B_ReadClassAttribute.vi", path "ClassProviders/Provider_EndevoGOOP300/Templates/BaseTemplate_4x4x4/methods/B_ReadProperty.vi", path "ClassProviders/Provider_EndevoGOOP300/Templates/BaseTemplate_4x4x4/methods/B_ReadWriteAttribute.vi", path "ClassProviders/Provider_EndevoGOOP300/Templates/BaseTemplate_4x4x4/methods/B_ReadWriteClassAttribute.vi", path "ClassProviders/Provider_EndevoGOOP300/Templates/BaseTemplate_4x4x4/methods/B_SetProperty.vi", path "ClassProviders/Provider_EndevoGOOP300/Templates/BaseTemplate_4x4x4/methods/B_WriteAttribute.vi", path "ClassProviders/Provider_EndevoGOOP300/Templates/BaseTemplate_4x4x4/methods/B_WriteClassAttribute.vi", path "ClassProviders/Provider_EndevoGOOP300/Templates/BaseTemplate_4x4x4/methods/B_WriteProperty.vi", path "ClassProviders/Provider_EndevoGOOP300/Templates/SubTemplate/methods/S_GetProperty.vi", path "ClassProviders/Provider_EndevoGOOP300/Templates/SubTemplate/methods/S_NoneModifing.vi", path "ClassProviders/Provider_EndevoGOOP300/Templates/SubTemplate/methods/S_ReadAttribute.vi", path "ClassProviders/Provider_EndevoGOOP300/Templates/SubTemplate/methods/S_ReadClassAttribute.vi", path "ClassProviders/Provider_EndevoGOOP300/Templates/SubTemplate/methods/S_ReadProperty.vi", path "ClassProviders/Provider_EndevoGOOP300/Templates/SubTemplate/methods/S_ReadWriteAttribute.vi", path "ClassProviders/Provider_EndevoGOOP300/Templates/SubTemplate/methods/S_ReadWriteClassAttribute.vi", path "ClassProviders/Provider_EndevoGOOP300/Templates/SubTemplate/methods/S_SetProperty.vi", path "ClassProviders/Provider_EndevoGOOP300/Templates/SubTemplate/methods/S_WriteAttribute.vi", path "ClassProviders/Provider_EndevoGOOP300/Templates/SubTemplate/methods/S_WriteClassAttribute.vi", path "ClassProviders/Provider_EndevoGOOP300/Templates/SubTemplate/methods/S_WriteProperty.vi", path "ClassProviders/Provider_EndevoGOOP300/Templates/SubTemplate_4x4x4/methods/S_GetProperty.vi", path "ClassProviders/Provider_EndevoGOOP300/Templates/SubTemplate_4x4x4/methods/S_NoneModifing.vi", path "ClassProviders/Provider_EndevoGOOP300/Templates/SubTemplate_4x4x4/methods/S_ReadAttribute.vi", path "ClassProviders/Provider_EndevoGOOP300/Templates/SubTemplate_4x4x4/methods/S_ReadClassAttribute.vi", path "ClassProviders/Provider_EndevoGOOP300/Templates/SubTemplate_4x4x4/methods/S_ReadProperty.vi", path "ClassProviders/Provider_EndevoGOOP300/Templates/SubTemplate_4x4x4/methods/S_ReadWriteAttribute.vi", path "ClassProviders/Provider_EndevoGOOP300/Templates/SubTemplate_4x4x4/methods/S_ReadWriteClassAttribute.vi", path "ClassProviders/Provider_EndevoGOOP300/Templates/SubTemplate_4x4x4/methods/S_SetProperty.vi", path "ClassProviders/Provider_EndevoGOOP300/Templates/SubTemplate_4x4x4/methods/S_WriteAttribute.vi", path "ClassProviders/Provider_EndevoGOOP300/Templates/SubTemplate_4x4x4/methods/S_WriteClassAttribute.vi", path "ClassProviders/Provider_EndevoGOOP300/Templates/SubTemplate_4x4x4/methods/S_WriteProperty.vi", path "SubVIs/CloneManyMethods.vi", path "SubVIs/GOOP_StartDebuggerController.vi", path "SubVIs/GOOP_StartObjectDebugger.vi", path "UML/ReversedEngineering/ReversedEngineering GetStateMachineCaseSelectorRefInfo.vit", path "UML/UMLEditor/UMLEditor TemplateObjectReference.ctt"]
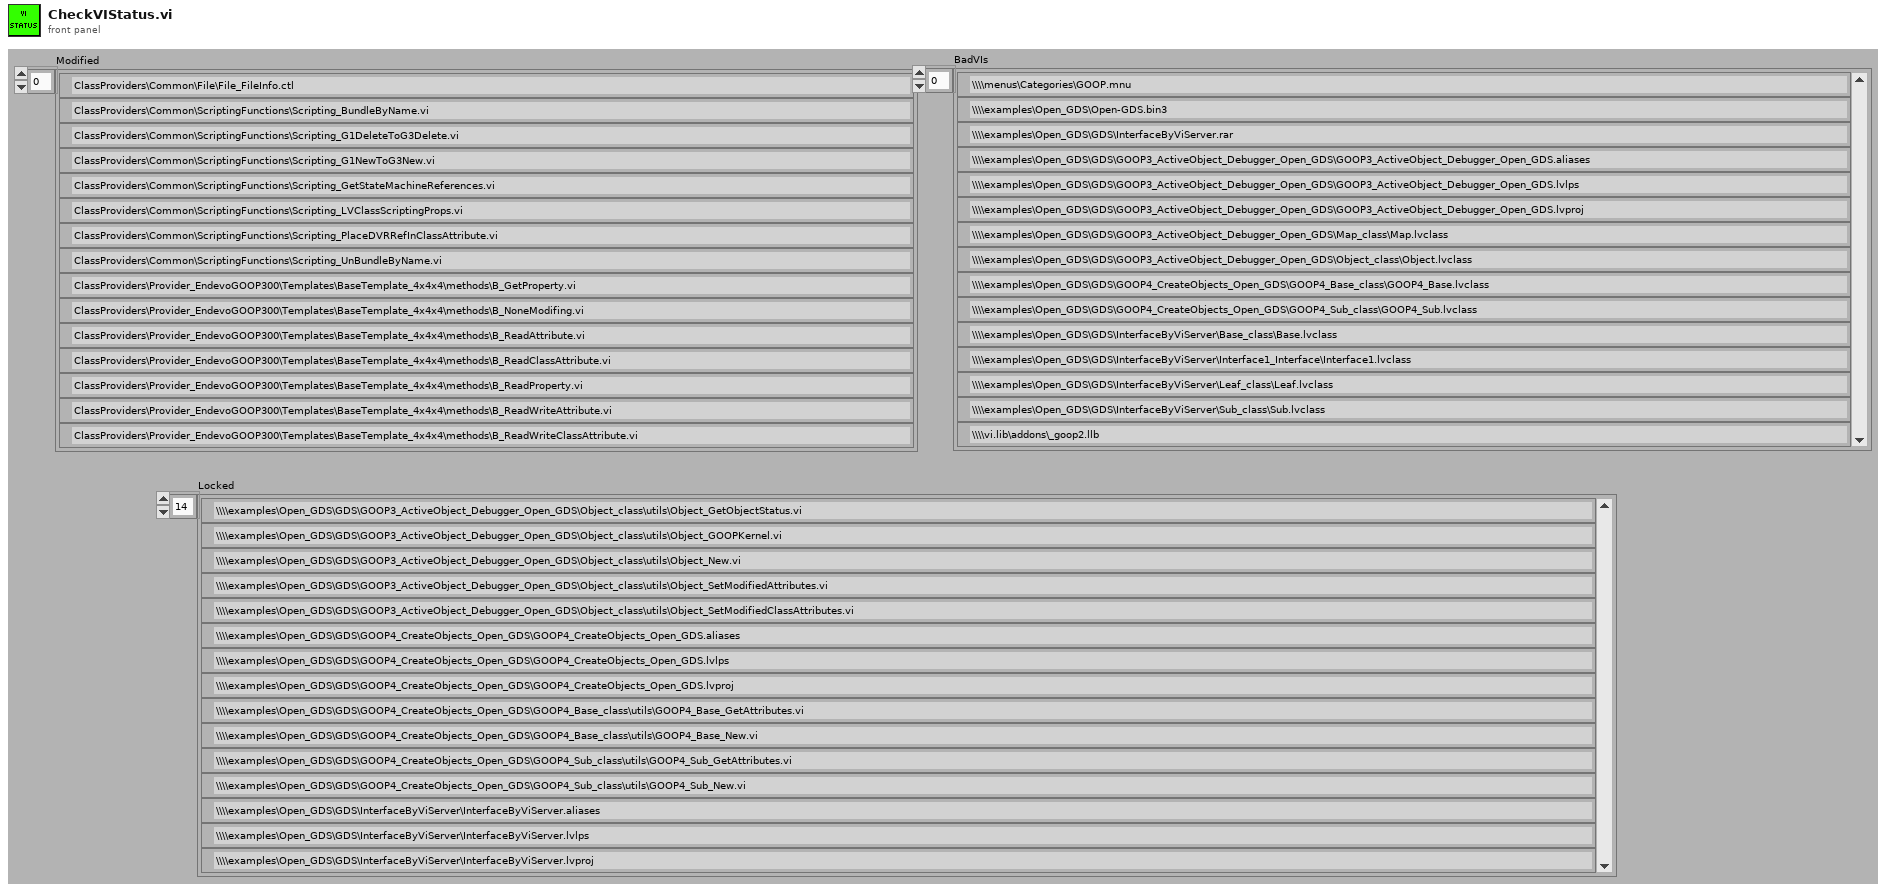
[diagram p1: front panel]
types:
  T1 = enum32{"Bad", "Idle", "Run top level", "Running"}
  T2 = enum32{"invalid lock state", "Not Locked", "Locked (No Password)", "Password-protected"}
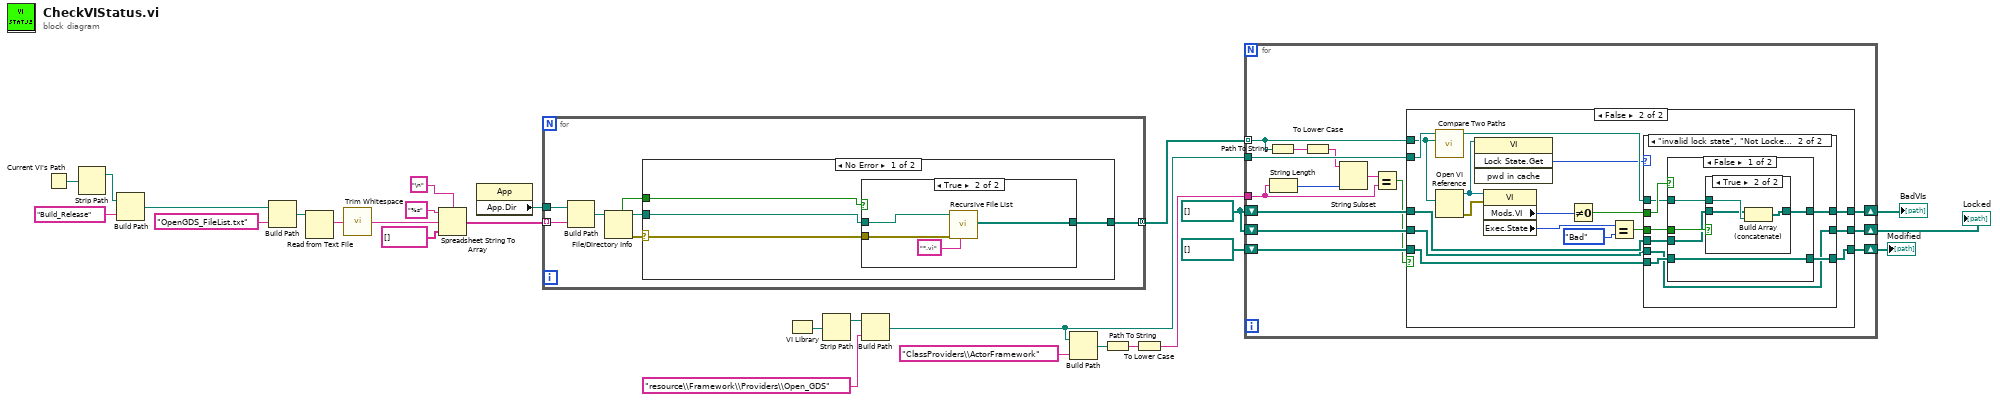
[diagram p0: block diagram]
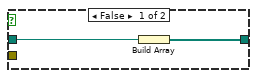
[diagram p2: hidden frame]
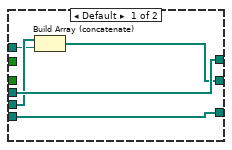
[diagram p5: hidden frame]
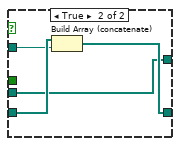
[diagram p7: hidden frame]
diagram:
  w3 = path[] []
  n1 = Current VI's Path() -> (path=w16:path)
  n2 = Strip Path(path=w16) -> (stripped path=w6:path)  [unwired: 1 out]
  n3 = Build Path(base path=w6, name or relative path="Build_Release") -> (appended path=w4:path)
  n4 = Build Path(base path=w4, name or relative path="OpenGDS_FileList.txt") -> (appended path=w13:path)
  n5 = Read from Text File(file (use dialog)=w13) -> (text=w12:string)  [unwired: 3 in, 3 out]
  n6 = call <vilib>:"Trim Whitespace.vi"("string"=w12) -> ("trimmed string"=w11:string)  [unwired: 1 in]
  n7 = Spreadsheet String To Array(delimiter (Tab)="\n", format string="%s", spreadsheet string=w11, array type (2D Dbl)=string[] []) -> (array=w7:string[])
  n8 = property class="App"() -> ("App.Dir"=w14:path)  [unwired: 2 in, 2 out]
  n9 = for {
    tunnel: w14 -> [w33]
    tunnel: w7 -> [w34] mode=indexing
    tunnel: [w28] -> w2 mode=concatenating
    n10 = Build Path(base path=w33, name or relative path=w34) -> (appended path=w32:path)
    n11 = File/Directory Info(path=w32) -> (path out=w29:path, directory=w30:bool, error out=w31:errorcluster)  [unwired: 1 in, 4 out]
    n12 = case shown="No Error" w31 {
      selector: w31 -> [w36 _]
      tunnel: w30 -> [w38 _]
      tunnel: w29 -> [w37 _]
      tunnel: [w35 _] -> w28
      frame No Error {
        n13 = case shown="True" w38 {
          tunnel: w37 -> [w40 w44]
          tunnel: w36 -> [_ w43]
          tunnel: [w39 w42] -> w35
          frame False {
            n14 = Build Array(w40) -> (w39:path[])
          }
          frame True {
            n15 = call <vilib>:"Recursive File List.vi"("pattern"="*.vi", "error in (no error)"=w43, "Folder Path"=w44) -> ("All Files in Dir"=w42:path[])  [unwired: 4 in, 4 out]
          }
        }
      }
      frame Error {
      }
    }
  }
  n16 = VI Library() -> (path=w27:path)
  n17 = Strip Path(path=w27) -> (stripped path=w26:path)  [unwired: 1 out]
  n18 = Build Path(base path=w26, name or relative path="resource\\Framework\\Providers\\Open_GDS") -> (appended path=w17:path)
  n19 = Build Path(base path=w17, name or relative path="ClassProviders\\ActorFramework") -> (appended path=w22:path)
  n20 = Path To String(path=w22) -> (string=w23:string)
  n21 = To Lower Case(string=w23) -> (all lower case string=w21:string)
  n22 = for {
    tunnel: w2 -> [w58] mode=indexing
    tunnel: w21 -> [w48]
    shift-right: [w56] -> w18
    shift-left: w3 -> [w57]
    shift-right: [w55] -> w19
    shift-left: path[] [] -> [w54]
    tunnel: w17 -> [w53]
    shift-right: [w46] -> w1
    shift-left: w3 -> [w47]
    n23 = Path To String(path=w58) -> (string=w52:string)
    n24 = String Length(string=w48) -> (length=w50:i32)
    n25 = To Lower Case(string=w52) -> (all lower case string=w51:string)
    n26 = String Subset(string=w51, length (rest)=w50) -> (substring=w49:string)  [unwired: 1 in]
    n27 = Equal?(x=w49, y=w48) -> (x = y?=w45:bool)
    n28 = case shown="False" w45 {
      tunnel: w58 -> [_ w67]
      tunnel: w57 -> [w61 w72]
      tunnel: [w61 w71] -> w56
      tunnel: w54 -> [w60 w69]
      tunnel: [w60 w70] -> w55
      tunnel: w53 -> [_ w68]
      tunnel: w47 -> [w59 w63]
      tunnel: [w59 w62] -> w46
      frame True {
      }
      frame False {
        n29 = call <vilib>:"Compare Two Paths.vi"("Path 2"=w67, "Path 1"=w68) -> ("Relative Path from 1 to 2"=w66:path)  [unwired: 6 in, 3 out]
        n30 = Open VI Reference(vi path=w67) -> (vi reference=w65:refnum<vi>, error out=w78:errorcluster)  [unwired: 5 in]
        n31 = invoke class="VI" method="Lock State.Get"(reference=w65) -> ("Get Lock State"=w64:T2)  [unwired: 3 in, 3 out]
        n32 = property class="VI"(reference=w65, error in=w78) -> ("Mods.VI"=w77:u64, "Exec.State"=w76:T1)  [unwired: 2 out]
        n33 = Not Equal To 0?(x=w77) -> (x != 0?=w74:bool)
        n34 = Equal?(x=w76, y=T1."Bad") -> (x = y?=w73:bool)
        n35 = case shown="\"invalid lock state\", \"Not Locked\"" w64 {
          tunnel: w74 -> [_ w91]
          tunnel: w73 -> [_ w90]
          tunnel: w72 -> [w82 w89]
          tunnel: [w82 w88] -> w71
          tunnel: [w83 w87] -> w70
          tunnel: w69 -> [w83 w86]
          tunnel: w66 -> [w79 w85]
          tunnel: w63 -> [w81 w84]
          tunnel: [w80 w84] -> w62
          frame Default {
            n36 = Build Array (concatenate)(w81, w79) -> (w80:path[])
          }
          frame "invalid lock state", "Not Locked" {
            n37 = case shown="False" w91 {
              tunnel: w90 -> [w96 _]
              tunnel: w85 -> [w95 w102]
              tunnel: w89 -> [w94 w101]
              tunnel: [w93 w101] -> w88
              tunnel: w86 -> [w92 w104]
              tunnel: [w92 w103] -> w87
              frame False {
                n38 = case shown="True" w96 {
                  tunnel: w95 -> [_ w100]
                  tunnel: w94 -> [w97 w99]
                  tunnel: [w97 w98] -> w93
                  frame False {
                  }
                  frame True {
                    n39 = Build Array (concatenate)(w99, w100) -> (w98:path[])
                  }
                }
              }
              frame True {
                n40 = Build Array (concatenate)(w104, w102) -> (w103:path[])
              }
            }
          }
        }
      }
    }
  }
  "Modified" <- w19
  "BadVIs" <- w18
  "Locked" <- w1
